vi "Strip Quotes and Unescape.vi"(8 "error in (no error)":errorcluster, 11 "String":string) -> (0 "error out":errorcluster, 3 "result string":string)   [LabVIEW 2019, in "JSONtext.lvlib"]
uses:
  JSONtext.lvlib
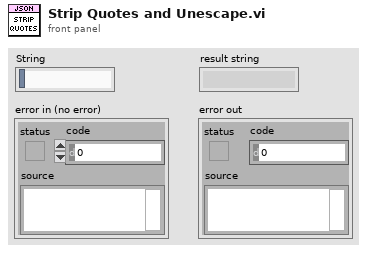
[diagram p1: front panel]
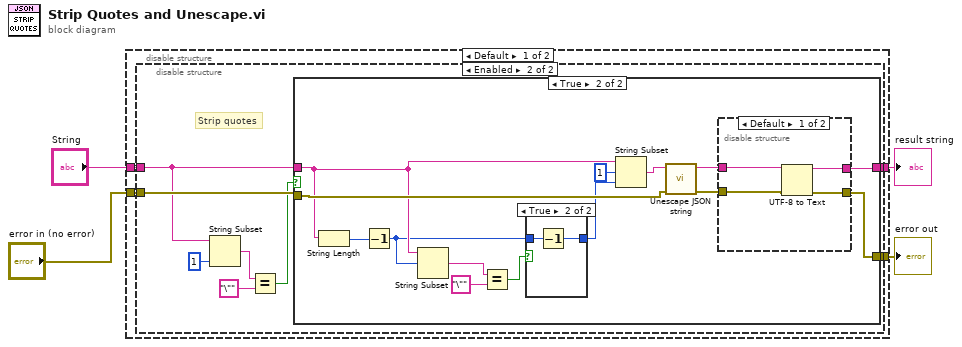
[diagram p0: block diagram]
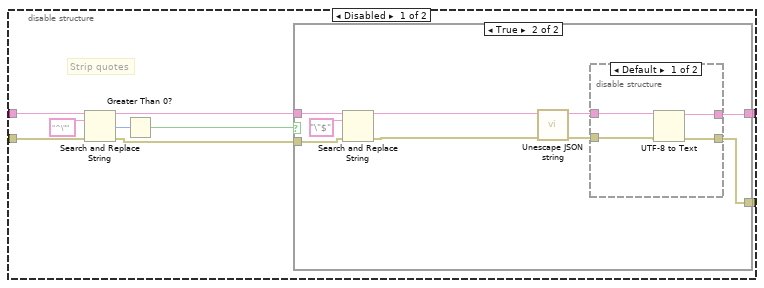
[diagram p2: hidden frame]
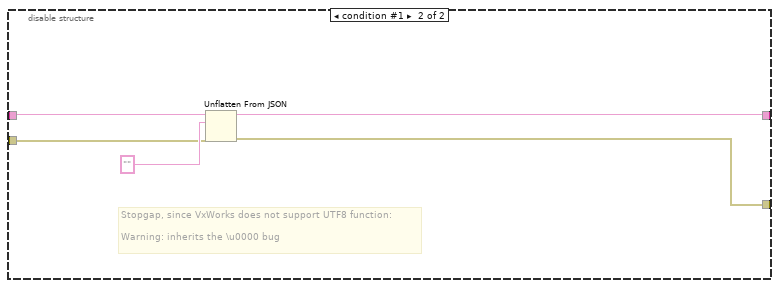
[diagram p8: hidden frame]
diagram:
  n1 = disable-structure shown="Default" {
    disable-tunnel: [w8 w68] -> w4
    disable-tunnel: "error in (no error)" -> [w7 w70]
    disable-tunnel: [w6 w69] -> w2
    disable-tunnel: "String" -> [w5 w72]
    frame condition #0 (active) {
      n2 = disable-structure shown="Enabled" {
        disable-tunnel: [w17 w42] -> w8
        disable-tunnel: w7 -> [w15 w41]
        disable-tunnel: [w14 w40] -> w6
        disable-tunnel: w5 -> [w9 w38]
        frame Disabled {
          # "Strip quotes"
          n3 = Search and Replace String(input string=w9, search string="^\"", error in=w15) -> (result string=w13:string, number of replacements=w11:i32, error out=w16:errorcluster)  [unwired: 5 in, 1 out]
          n4 = Greater Than 0?(x=w11) -> (x > 0?=w10:bool)
          n5 = case shown="True" w10 {
            tunnel: [w18 w20] -> w17
            tunnel: w16 -> [w18 w28]
            tunnel: [w19 w22] -> w14
            tunnel: w13 -> [w19 w27]
            frame False {
              # "Not a leading quote?   This shouldn't happen."
            }
            frame True {
              n6 = Search and Replace String(input string=w27, search string="\"$", error in=w28) -> (result string=w25:string, error out=w24:errorcluster)  [unwired: 5 in, 2 out]
              n7 = call "Unescape JSON string.vi"("error in (no error)"=w24, "Text (with JSON escapes)"=w25) -> ("error out"=w21:errorcluster, "Text (unescaped)"=w23:string)  [unwired: 8 in]
              n8 = disable-structure shown="Default" {
                disable-tunnel: w23 -> [w32 w34]
                disable-tunnel: [w31 w34] -> w22
                disable-tunnel: w21 -> [w30 w33]
                disable-tunnel: [w29 w33] -> w20
                frame condition #0 (active) {
                  n9 = UTF-8 to Text(8:w30, 11:w32) -> (0:w29:errorcluster, 3:w31:string)  [unwired: 1 in]
                }
                frame condition #1 {
                }
              }
            }
          }
        }
        frame Enabled {
          # "Strip quotes"
          n10 = String Subset(string=w38, length (rest)=1 ("length (rest)")) -> (substring=w37:string)  [unwired: 1 in]
          n11 = Equal?(x=w37, y="\"") -> (x = y?=w35:bool)
          n12 = case shown="True" w35 {
            tunnel: [w43 w54] -> w42
            tunnel: w41 -> [w43 w58]
            tunnel: [w44 w56] -> w40
            tunnel: w38 -> [w44 w50]
            frame False {
            }
            frame True {
              n13 = String Length(string=w50) -> (length=w51:i32)
              n14 = Decrement(x=w51) -> (x-1=w47:i32)
              n15 = String Subset(string=w50, offset (0)=w47) -> (substring=w52:string)  [unwired: 1 in]
              n16 = Equal?(x=w52, y="\"") -> (x = y?=w45:bool)
              n17 = case shown="True" w45 {
                tunnel: w47 -> [w59 w61]
                tunnel: [w59 w60] -> w46
                frame False {
                }
                frame True {
                  n18 = Decrement(x=w61) -> (x-1=w60:i32)
                }
              }
              n19 = String Subset(string=w50, offset (0)=1, length (rest)=w46) -> (substring=w48:string)
              n20 = call "Unescape JSON string.vi"("error in (no error)"=w58, "Text (with JSON escapes)"=w48) -> ("error out"=w55:errorcluster, "Text (unescaped)"=w57:string)  [unwired: 8 in]
              n21 = disable-structure shown="Default" {
                disable-tunnel: w57 -> [w65 w67]
                disable-tunnel: [w64 w67] -> w56
                disable-tunnel: w55 -> [w63 w66]
                disable-tunnel: [w62 w66] -> w54
                frame condition #0 (active) {
                  n22 = UTF-8 to Text(8:w63, 11:w65) -> (0:w62:errorcluster, 3:w64:string)  [unwired: 1 in]
                }
                frame condition #1 {
                }
              }
            }
          }
        }
      }
    }
    frame condition #1 {
      # "Stopgap, since VxWorks does not support UTF8 function:\n\nWarning: inherits the \\u0000 bug"
      n23 = Unflatten From JSON(JSON string=w72, type and defaults="", error in (no error)=w70) -> (value=w69:string, error out=w68:errorcluster)  [unwired: 4 in]
    }
  }
  "error out" <- w4
  "result string" <- w2
